vi "Periodic Tasks.vi"(8 "error in":errorcluster) -> ()   [LabVIEW 2019]
doc: "This VI runs in parallel to other tasks. It can contain as many user-defined periodic loops as you need. These can carry out PID or other sorts of timed response."
uses:
  <vilib>/Rock Robotics/Network Tables/NT Write Number.vi
  <vilib>/Rock Robotics/Network Tables/NT Write Numeric Array.vi
  Robot Global Data.vi
  <vilib>/Rock Robotics/Network Tables/NT Read Number.vi
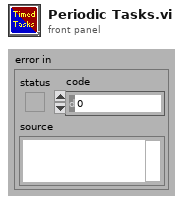
[diagram p1: front panel]
types:
  T1 = typedef "WPI_JoystickDevRef.ctl" = cluster{"Device":T2}
  T2 = typedef "WPI_JoystickDeviceEnum.ctl" = enum16{"USB 0", "USB 1", "USB 2", "USB 3", "USB 4", "USB 5"}
  T3 = typedef "WPI_RobotDriveDevRef.ctl" = cluster{"DevStatus":errorcluster, "Motors[]":T4[], "Square Inputs":bool, "Max Output":dbl}
  T4 = typedef "WPI_MotorControlDeviceRef.ctl" = cluster{"DeviceStatus":errorcluster, "Type":T5, "PWM":cluster{"PWM Channel":T6, "DeadBand":T7}, "CAN":cluster{"Device Number":u8, "SetOutput VI Ref":variant, "GetOutput VI Ref":variant, "Enable VI Ref":variant, "Disable VI Ref":variant, "Data":variant}, "Invert":bool, "DIO PWM":cluster{"PWM \"Enable\" Channel":T6, "DIOChannel":T8, "PWM Rate":dbl}}
  T5 = typedef "WPI_MotorControlType.ctl" = enum16{"PWM", "CAN", "DIO PWM"}
  T6 = typedef "FPGA_DIOPWMChannel.ctl" = enum8{"PWM 0", "PWM 1", "PWM 2", "PWM 3", "PWM 4", "PWM 5", "PWM 6", "PWM 7", "PWM 8", "PWM 9", "PWM MXP 0", "PWM MXP 1", "PWM MXP 2", "PWM MXP 3", "PWM MXP 4", "PWM MXP 5", "PWM MXP 6", "PWM MXP 7", "PWM MXP 8", "PWM MXP 9", "Invalid"}
  T7 = typedef "WPI_PWMDeadband.ctl" = cluster{"Name":string, "maxPositivePwm":i32, "minPositivePwm":i32, "centerPwm":i32, "maxNegativePwm":i32, "minNegativePwm":i32, "angularRange":u16}
  T8 = typedef "FPGA_DIOChannel.ctl" = enum8{"DIO 0", "DIO 1", "DIO 2", "DIO 3", "DIO 4", "DIO 5", "DIO 6", "DIO 7", "DIO 8", "DIO 9", "DIO MXP 0", "DIO MXP 1", "DIO MXP 2", "DIO MXP 3", "DIO MXP 4", "DIO MXP 5", "DIO MXP 6", "DIO MXP 7", "DIO MXP 8", "DIO MXP 9", "DIO MXP 10", "DIO MXP 11", "DIO MXP 12", "DIO MXP 13", "DIO MXP 14", "DIO MXP 15", "SPI Port CS1", "SPI Port CS2", "SPI Port CS3", "SPI Port MISO", "SPI Port MOSI", "Invalid"}
  T9 = cluster{"JoystickDevRef":T1, "RobotDriveDevRef":T3}
  T10 = typedef "WPI_PotentiometerDevRef.ctl" = cluster{"DevStatus":errorcluster, "Analog Channel":T11, "Invert Output":bool}
  T11 = typedef "FPGA_AIChannel.ctl" = enum8{"AI 0", "AI 1", "AI 2", "AI 3", "AI MXP 0", "AI MXP 1", "AI MXP 2", "AI MXP 3", "Invalid"}
  T12 = typedef "WPI_AccelerometerDevRef.ctl" = cluster{"DevStatus":errorcluster, "Scaling":T13, "Analog Channels":T14, "I2C Bus":T15, "SPI Bus":T16, "Accel Range":T17, "ADXL Axes":T18, "Handle":i32, "Device Address":u8, "Accel Type":enum16{"Analog", "ADXL345 I2C", "ADXL345 SPI", "Internal", "ADXL362 SPI"}}
  T13 = typedef "WPI_AccelerometerScaling.ctl" = cluster{"Gain (VoltsPerG)":dbl, "Center Voltage":dbl}
  T14 = typedef "WPI_AccelerometerAnalogChannels.ctl" = cluster{"X-Axis":T11, "Y-Axis":T11, "Z-Axis":T11}
  T15 = typedef "i2c_bus.ctl" = enum16{"I2C On-Board", "I2C MXP", "Invalid"}
  T16 = typedef "spi_bus.ctl" = enum16{"SPI On-Board, CS0", "SPI On-Board, CS1", "SPI On-Board, CS2", "SPI On-Board, CS3", "SPI MXP", "Invalid"}
  T17 = typedef "ADXL345 Range.ctl" = u8
  T18 = typedef "WPI_AccelerometerADXL345 Axes.ctl" = cluster{"X-Axis":bool, "Y-Axis":bool, "Z-Axis":bool}
  T19 = cluster{"X-Axis":dbl, "Y-Axis":dbl, "Z-Axis":dbl}
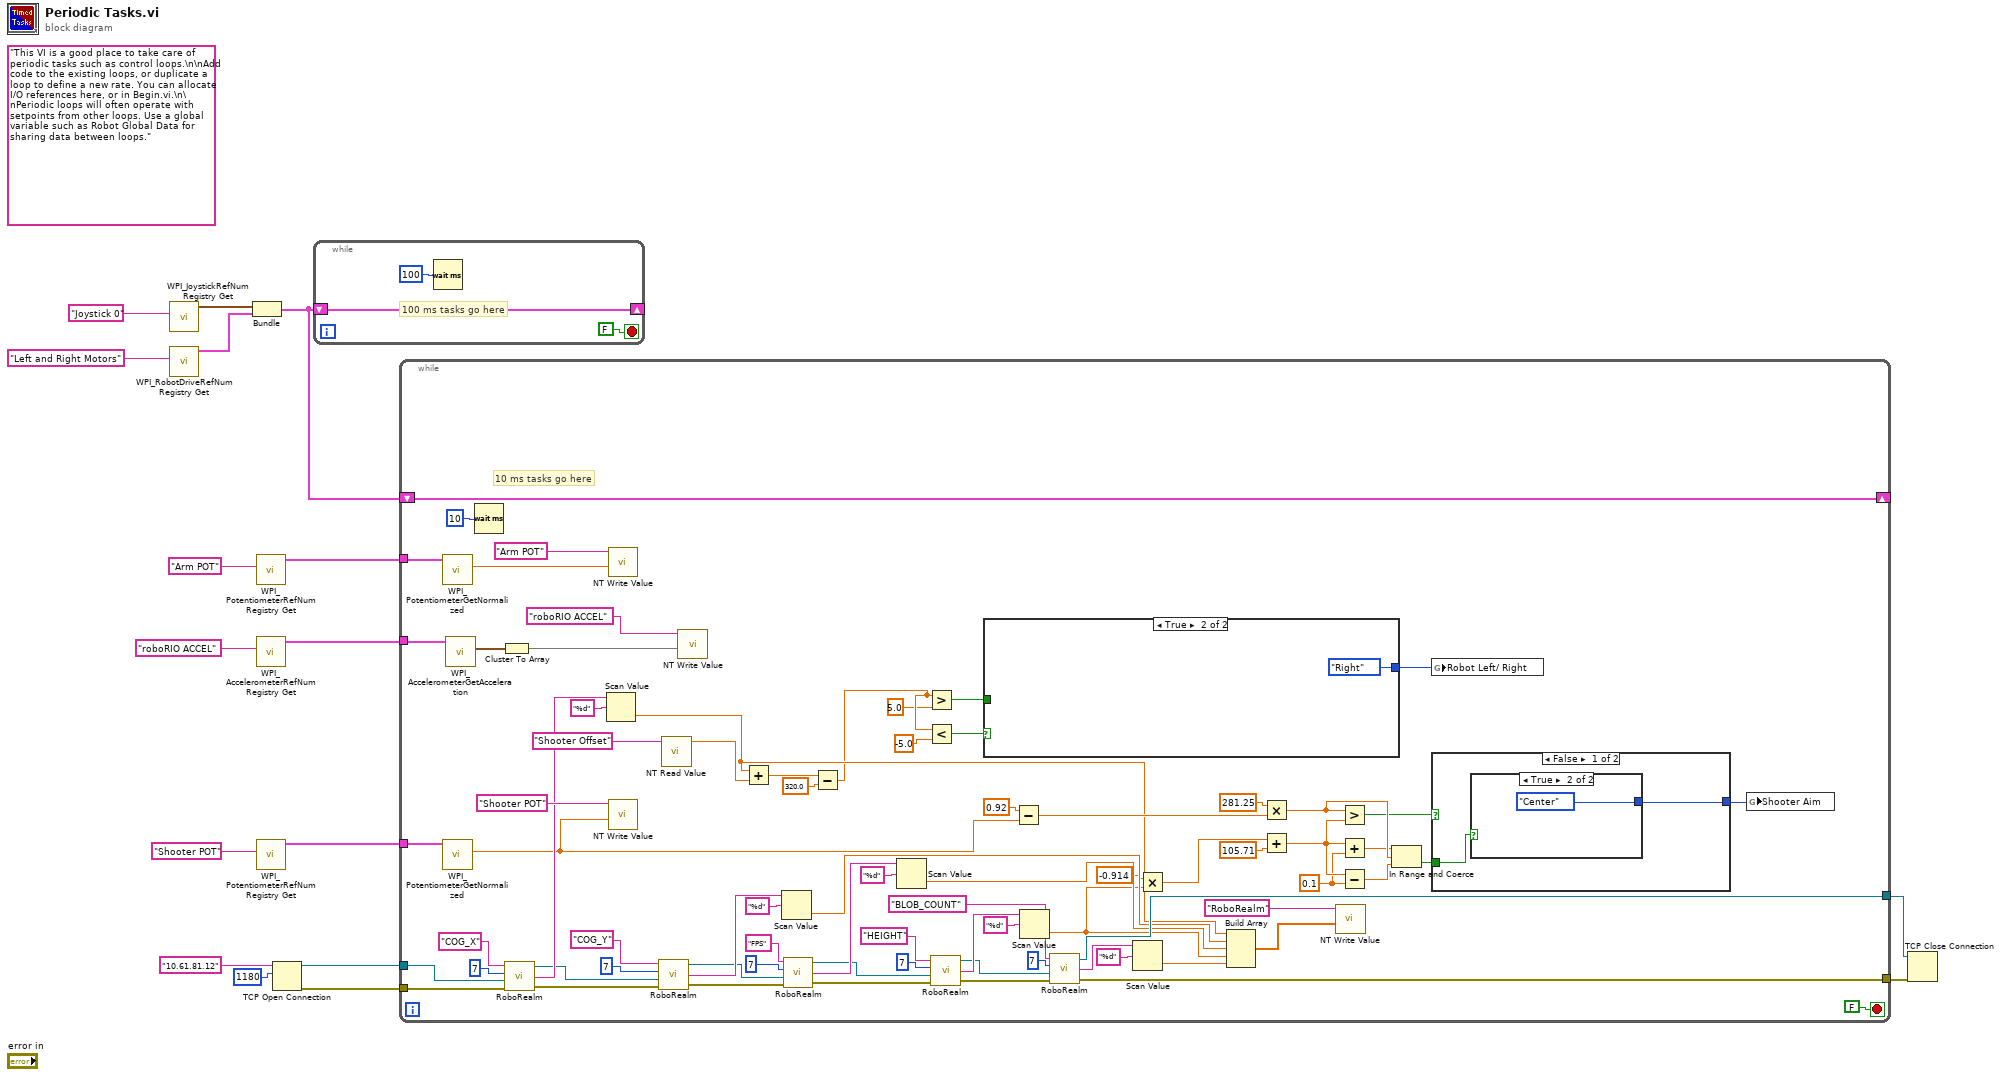
[diagram p0: block diagram]
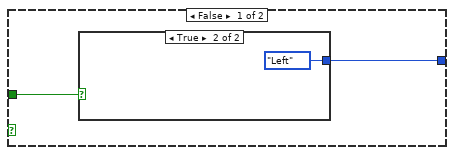
[diagram p2: hidden frame]
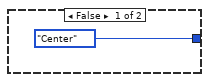
[diagram p3: hidden frame]
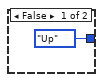
[diagram p4: hidden frame]
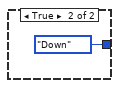
[diagram p5: hidden frame]
diagram:
  (unwired) "This VI is a good place to take care of periodic tasks such as control loops.\n\nAdd code to the existing loops, or duplicate a loop to define a new rate. You can allocate I/O references here, or in Begin.vi.\n\nPeriodic loops will often operate with setpoints from other loops. Use a global variable such as Robot Global Data for sharing data between loops."
  n1 = call <vilib>:"WPI_JoystickRefNum Registry Get.vi"("refnum name"="Joystick 0") -> ("JoystickDevRef"=w15:T1)  [unwired: 1 in, 9 out]
  n2 = call <vilib>:"WPI_RobotDriveRefNum Registry Get.vi"("refnum name"="Left and Right Motors") -> ("RobotDriveDevRef"=w14:T3)  [unwired: 1 in, 9 out]
  n3 = Bundle("JoystickDevRef"=w15, "RobotDriveDevRef"=w14) -> (w13:T9)  [unwired: 1 out]
  n4 = call <vilib>:"WPI_PotentiometerRefNum Registry Get.vi"("refnum name"="Arm POT") -> ("PotDevRef"=w9:T10)  [unwired: 9 in, 1 out]
  n5 = call <vilib>:"WPI_AccelerometerRefNum Registry Get.vi"("refnum name"="roboRIO ACCEL") -> ("AccelerometerDevRef"=w7:T12)  [unwired: 9 in, 1 out]
  n6 = call <vilib>:"WPI_PotentiometerRefNum Registry Get.vi"("refnum name"="Shooter POT") -> ("PotDevRef"=w10:T10)  [unwired: 9 in, 1 out]
  n7 = TCP Open Connection(address="10.61.81.12", remote port or service name=u16 1180) -> (connection ID=w4:refnum<k5>, error out=w1:errorcluster)  [unwired: 3 in]
  n8 = while {
    shift-right: [w18] -> _
    shift-left: w13 -> [w18]
    stop <- FALSE stop-if-true
    # "100 ms tasks go here"
    n9 = Wait (ms)(milliseconds to wait=u32 100) -> ()  [unwired: 1 out]
  }
  n10 = while {
    shift-right: [w94] -> _
    shift-left: w13 -> [w94]
    tunnel: w10 -> [w90]
    tunnel: w9 -> [w89]
    tunnel: w7 -> [w88]
    tunnel: w4 -> [w56]
    tunnel: [w55] -> w3
    tunnel: [w54] -> w2
    tunnel: w1 -> [w53]
    stop <- FALSE stop-if-true
    w35 = 0.1 ("y")
    # "10 ms tasks go here"
    n11 = call <vilib>:"WPI_PotentiometerGetNormalized.vi"("PotDevRef"=w89) -> ("Normalized Value"=w92:dbl)  [unwired: 8 in, 2 out]
    n12 = call <vilib>:"WPI_PotentiometerGetNormalized.vi"("PotDevRef"=w90) -> ("Normalized Value"=w40:dbl)  [unwired: 8 in, 2 out]
    n13 = call <vilib>:"WPI_AccelerometerGetAcceleration.vi"("AccelerometerDevRef"=w88) -> ("Accelerations"=w87:T19)  [unwired: 8 in, 2 out]
    n14 = Wait (ms)(milliseconds to wait=u32 10) -> ()  [unwired: 1 out]
    n15 = Cluster To Array(cluster=w87) -> (array=w86:dbl[])
    n16 = call "RoboRealm.vi"("error in (no error)"=w53, "connection ID IN"=w56, "Max Variable Length"=7, "Variable Name"="COG_X") -> ("error out"=w58:errorcluster, "Variable Value"=w82:string, "connection ID out"=w71:refnum<k5>)
    n17 = Scan Value(string=w82, format string="%d") -> (value=w30:dbl)  [unwired: 1 in, 1 out]
    n18 = call-poly <vilib>:"NT Write Value.vi"("Numeric"=w92, "Name"="Arm POT") -> ()  [unwired: 9 in, 1 out]
    n19 = call-poly <vilib>:"NT Write Value.vi"("Numeric"=w40, "Name"="Shooter POT") -> ()  [unwired: 9 in, 1 out]
    n20 = call "RoboRealm.vi"("error in (no error)"=w58, "connection ID IN"=w71, "Max Variable Length"=7, "Variable Name"="COG_Y") -> ("error out"=w57:errorcluster, "Variable Value"=w79:string, "connection ID out"=w72:refnum<k5>)
    n21 = call-poly <vilib>:"NT Read Value.vi"("Name"="Shooter Offset") -> ("Numeric"=w28:dbl)  [unwired: 9 in, 1 out]
    n22 = call-poly <vilib>:"NT Write Value.vi"("Numeric Array"=w86, "Name"="roboRIO ACCEL") -> ()  [unwired: 9 in, 1 out]
    n23 = Add(x=w30, y=w28) -> (x+y=w29:dbl)
    n24 = Scan Value(string=w79, format string="%d") -> (value=w52:dbl)  [unwired: 1 in, 1 out]
    n25 = call "RoboRealm.vi"("error in (no error)"=w57, "connection ID IN"=w72, "Max Variable Length"=7, "Variable Name"="FPS") -> ("error out"=w60:errorcluster, "Variable Value"=w74:string, "connection ID out"=w62:refnum<k5>)
    n26 = Subtract(x=w29, y=320.0) -> (x-y=w23:dbl)
    n27 = Scan Value(string=w74, format string="%d") -> (value=w51:dbl)  [unwired: 1 in, 1 out]
    n28 = Greater?(x=w23, y=5.0) -> (0:w25:bool)
    n29 = Less?(x=w23, y=-5.0) -> (x < y?=w26:bool)
    n30 = call "RoboRealm.vi"("error in (no error)"=w60, "connection ID IN"=w62, "Max Variable Length"=7, "Variable Name"="HEIGHT") -> ("error out"=w59:errorcluster, "Variable Value"=w69:string, "connection ID out"=w61:refnum<k5>)
    n31 = case shown="True" w26 {
      tunnel: w25 -> [w98 _]
      tunnel: [w97 enum16{"Left", "Right", "Center"}."Right" ("Robot Left/ Right")] -> w24
      frame False {
        n32 = case shown="True" w98 {
          tunnel: [enum16{"Left", "Right", "Center"}."Center" ("Robot Left/ Right") enum16{"Left", "Right", "Center"}."Left" ("Robot Left/ Right")] -> w97
          frame False {
          }
          frame True {
          }
        }
      }
      frame True {
      }
    }
    n33 = Subtract(x=0.92, y=w40) -> (x-y=w42:dbl)
    n34 = Scan Value(string=w69, format string="%d") -> (value=w45:dbl)  [unwired: 1 in, 1 out]
    n35 = call "RoboRealm.vi"("error in (no error)"=w59, "connection ID IN"=w61, "Max Variable Length"=7, "Variable Name"="BLOB_COUNT") -> ("error out"=w54:errorcluster, "Variable Value"=w64:string, "connection ID out"=w55:refnum<k5>)
    n36 = Scan Value(string=w64, format string="%d") -> (value=w50:dbl)  [unwired: 1 in, 1 out]
    n37 = Multiply(x=-0.914, y=w45) -> (x*y=w47:dbl)
    n38 = Build Array(w30, w52, w51, w45, w50) -> (w49:dbl[])
    n39 = Multiply(x=281.25, y=w42) -> (x*y=w39:dbl)
    n40 = Add(x=w47, y=105.71) -> (x+y=w36:dbl)
    n41 = call-poly <vilib>:"NT Write Value.vi"("Numeric Array"=w49, "Name"="RoboRealm") -> ()  [unwired: 9 in, 1 out]
    n42 = Greater?(x=w39, y=w36) -> (0:w33:bool)
    n43 = Add(x=w36, y=w35) -> (x+y=w38:dbl)
    n44 = Subtract(x=w36, y=w35) -> (x-y=w37:dbl)
    n45 = In Range and Coerce(upper limit=w38, x=w39, lower limit=w37) -> (In Range?=w34:bool)  [unwired: 1 out]
    n46 = global write "Robot Global Data.vi" "Robot Left/ Right"(w24) -> ()
    n47 = case shown="False" w33 {
      tunnel: w34 -> [w103 _]
      tunnel: [w102 enum16{"Up", "Down", "Center"}."Down"] -> w32
      frame False {
        n48 = case shown="True" w103 {
          tunnel: [enum16{"Up", "Down", "Center"}."Up" enum16{"Up", "Down", "Center"}."Center"] -> w102
          frame False {
          }
          frame True {
          }
        }
      }
      frame True {
      }
    }
    n49 = global write "Robot Global Data.vi" "Shooter Aim"(w32) -> ()
  }
  n50 = TCP Close Connection(connection ID=w3, error in (no error)=w2) -> ()  [unwired: 1 in, 2 out]
